vi "De-queue RT FIFO loop element.vi"(11 "RT Queues":T1) -> (0 "Data":variant, 2 "Message":string, 3 "timed out?":bool, 4 "remaining queue elements":i32)   [LabVIEW 2018]
uses:
  Type Defs/Queues cluster.ctl
  ICL-LabVIEW_General/Message Scheduler/message scheduler.lvclass
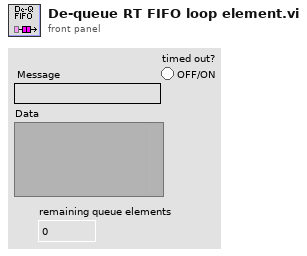
[diagram p1: front panel]
types:
  T1 = typedef "Queues cluster.ctl" = cluster{"RT Message":refnum<queue>, "RT Comms":refnum<queue>, "RT Data":refnum<queue>, "RT FIFO":refnum<queue>, "message scheduler":refnum<class "message scheduler.lvclass">}
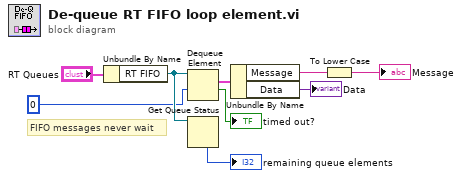
[diagram p0: block diagram]
diagram:
  # "FIFO messages never wait"
  n1 = Unbundle By Name("RT Queues") -> ("RT FIFO"=w4:refnum<queue>)
  n2 = Dequeue Element(queue=w4, timeout in ms (-1)=0) -> (element=w8:cluster{"Message":string, "Data":variant}, timed out?=→"timed out?":bool)  [unwired: 1 in, 2 out]
  n3 = Get Queue Status(queue=w4) -> (# elements in queue=→"remaining queue elements":i32)  [unwired: 2 in, 7 out]
  n4 = Unbundle By Name(w8) -> ("Message"=w7:string, "Data"=→"Data":variant)
  n5 = To Lower Case(string=w7) -> (all lower case string=→"Message":string)
